vi "19.1.1-Meter Reader.vi"() -> ()   [LabVIEW 2017]
doc: "This example shows how to compute the histogram of an image or a region in the image. This example also shows how to set up and use the display tools to select and work on different regions in the image interactively."
uses:
  <vilib>/vision/NI_Vision_Development_Module.lvlib
panel:
  out "Results:":dbl format="%#_2g"
  out "Image":T1(plugin-control)
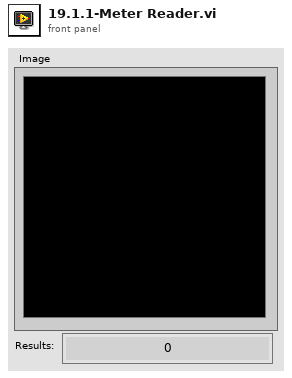
[diagram p1: front panel]
types:
  T1 = typedef "IMAQ Image.ctl" = refnum<image>
  T2 = typedef "Image Type" = u32
  T3 = typedef "IMAQ Line" = cluster{"Start X":i32, "Start Y":i32, "End X":i32, "End Y":i32}
  T4 = typedef "ROI Descriptor" = cluster{"Global Rectangle":i32[], "Contours":cluster{"ID":enum32{"External", "Internal"}, "Type":u32, "Coordinates":i32[]}[]}
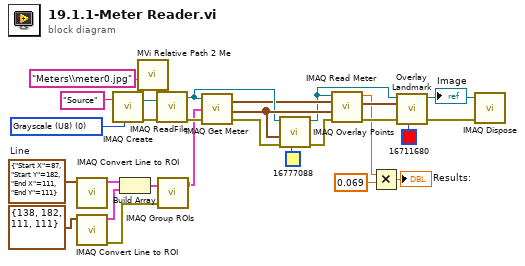
[diagram p0: block diagram]
diagram:
  w18 = T2 0 items=["Grayscale (U8)", "Grayscale (I16)", "Grayscale (SGL)", "Complex (CSG)", "RGB (U32)", "HSL (U32)", "RGB (U64)", "Grayscale (U16)"] ("Image Type")
  w20 = T3 {"Start X"=87, "Start Y"=182, "End X"=111, "End Y"=111}  # Line
  n1 = call "IMAQ Convert Line to ROI"("Line"=w20) -> ("ROI Descriptor"=w24:T4)  [unwired: 8 in, 1 out]
  n2 = call "IMAQ Convert Line to ROI"("Line"=T3 {"Start X"=138, "Start Y"=182, "End X"=111, "End Y"=111}) -> ("error out"=w21:errorcluster, "ROI Descriptor"=w23:T4)  [unwired: 8 in]
  n3 = call "IMAQ Create"("Image Name"="Source", "Image Type"=w18) -> ("New Image"=w29:T1, "error out"=w28:errorcluster)  [unwired: 3 in]
  n4 = Build Array(w24, w23) -> (w22:T4[])
  n5 = call "MVi Relative Path 2 Me.vi"("Relative Path"="Meters\\meter0.jpg") -> ("Appended Dir"=w26:path)  [unwired: 5 in, 1 out]
  n6 = call "IMAQ ReadFile"("File Path"=w26, "error in (no error)"=w28, "Image"=w29) -> ("error out"=w17:errorcluster, "Image Out"=w10:T1)  [unwired: 4 in, 3 out]
  n7 = call "IMAQ Group ROIs"("error in (no error)"=w21, "ROI Descriptors"=w22) -> ("ROI Descriptor out"=w16:T4)  [unwired: 2 in, 1 out]
  n8 = call "IMAQ Get Meter"("Image"=w10, "ROI Descriptor"=w16, "error in (no error)"=w17) -> ("Needle Base"=w9:cluster{"X":sgl, "Y":sgl}, "Points Arc"=w14:cluster{"X":sgl, "Y":sgl}[], "error out"=w13:errorcluster)  [unwired: 4 in]
  n9 = call "IMAQ Overlay Points"("Color"=u32 16777088, "error in (no error)"=w13, "Array of Points"=w14, "Image"=w10) -> ("error out"=w12:errorcluster, "Image Out"=w5:T1)  [unwired: 6 in]
  n10 = call "IMAQ Read Meter"("error in (no error)"=w12, "Arc Points"=w14, "Needle Base"=w9, "Image"=w5) -> ("error out"=w8:errorcluster, "Point"=w6:cluster{"X":sgl, "Y":sgl}, "Percentage of scale"=w2:dbl)  [unwired: 5 in]
  n11 = Multiply(x=w2, y=0.069) -> (x*y=→"Results:":dbl)
  n12 = call "Overlay Landmark.vi"("Color"=u32 16711680, "error in"=w8, "Position"=w6, "Image"=w5) -> ("error out"=w7:errorcluster, "Image Out"=w3:T1)  [unwired: 6 in]
  "Image" <- w3
  n13 = call "IMAQ Dispose"("Image"=w3, "error in (no error)"=w7) -> ()  [unwired: 4 in, 1 out]
